vi "Main3.vi"() -> ()   [LabVIEW 2020]
uses:
  <vilib>/userDefined/High Color/IMAQdx.ctl
  <vilib>/vision/Image Controls.llb/IMAQ Image.ctl
  <vilib>/DAQmx/read.llb/DAQmx Read (Analog Wfm 1Chan NSamp).vi
  <vilib>/Utility/error.llb/Error Cluster From Error Code.vi
  <vilib>/DAQmx/miscellaneous.llb/DAQmx Fill In Error Info.vi
  <vilib>/ErrorRing/Error Ring.xnode
  SuportVI2/Message Queue/Message Queue.lvlib
  SuportVI2/User Event - Stop/User Event - Stop.lvlib
  <vilib>/vision/driver/NI_Vision_Acquisition_Software.lvlib
panel:
  out "XY Graph":cluster{dbl[], dbl[]}(graph)
  in  "Data":string="000001"
  in  "Is start":bool
  out "Waveform Graph":waveform(dbl)(graph)
  in  "Aquire Configuration":T1
  in  "Stop Acquire":bool
  in  "Start Acquire":bool
  in  "Stop SinusGen":bool
  in  "Start SinusGen":bool
  in  "Generator Configuration":T1
  out "Image":T2(plugin-control)
  in  "Camera Config":cluster{"Camera Select":T3}={"Camera Select"="cam0"}
  in  "Exit":bool
  in  "Stop Camera":bool
  in  "Start Camera":bool
  out "Status Line":string
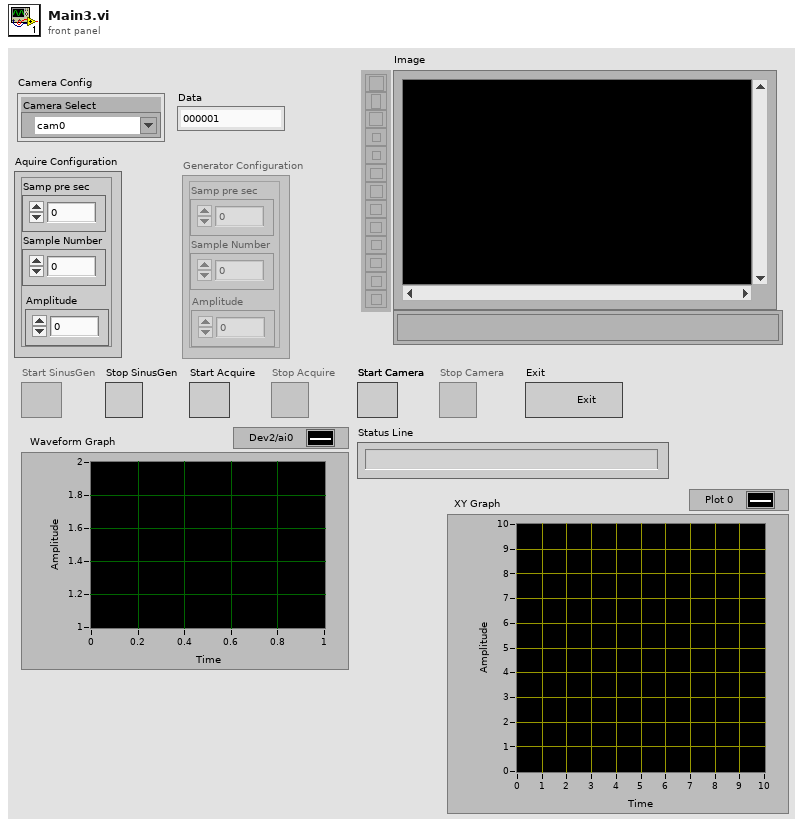
[diagram p1: front panel]
types:
  T1 = cluster{"Sample Number":dbl, "Samp pre sec":i32, "Amplitude":dbl}
  T2 = typedef "IMAQ Image.ctl" = refnum<image>
  T3 = typedef "IMAQdx.ctl" = refnum<k21>
  T4 = cluster{"configuration file path out":path, "DAQmx Task":refnum<k21>, "DAQmx Chanel":cluster{"SampClk.Rate":dbl, "SampQuant.SampPerChan":i32, "Amplitude 2":dbl}}
  T5 = cluster{"DAQmx Task":refnum<k21>, "DAQmx Chanel":cluster{"SampClk.Rate":dbl, "SampQuant.SampPerChan":i32, "Amplitude":dbl}, "DB Data":dbl[][], "DB Cuttoff":dbl[][]}
  T6 = cluster{"Image":cluster{"Image original":T2, "Image copy":T2, "Image Out":T2}, "Session Config":cluster{"Session":T3}, "Data":string}
  T7 = cluster{"Start Camera":refnum<vi>, "Stop Camera":refnum<vi>, "Exit":refnum<vi>, "Camera Conf":refnum<vi>, "Status Line":refnum<vi>, "Status Line Text":string, "Camera Select":refnum<vi>, "Start Acquire":refnum<vi>, "Stop Acquire":refnum<vi>, "Start SinusGen":refnum<vi>, "Stop SinusGen":refnum<vi>, "Generator Configuration":refnum<vi>, "Aquire Configuration":refnum<vi>}
  T8 = cluster{"UI":refnum<queue>, "Camera":refnum<queue>, "Acquire":refnum<queue>, "SinusGen":refnum<queue>}
  T9 = cluster{"SampClk.Rate":dbl, "SampQuant.SampPerChan":i32, dbl}
  T10 = cluster{"SampClk.Rate":dbl, "SampQuant.SampPerChan":i32, "Amplitude":dbl}
  T11 = typedef "Image Type" = u32
  T12 = cluster{"SampClk.Rate":dbl, "SampQuant.SampPerChan":i32, "Amplitude 2":dbl}
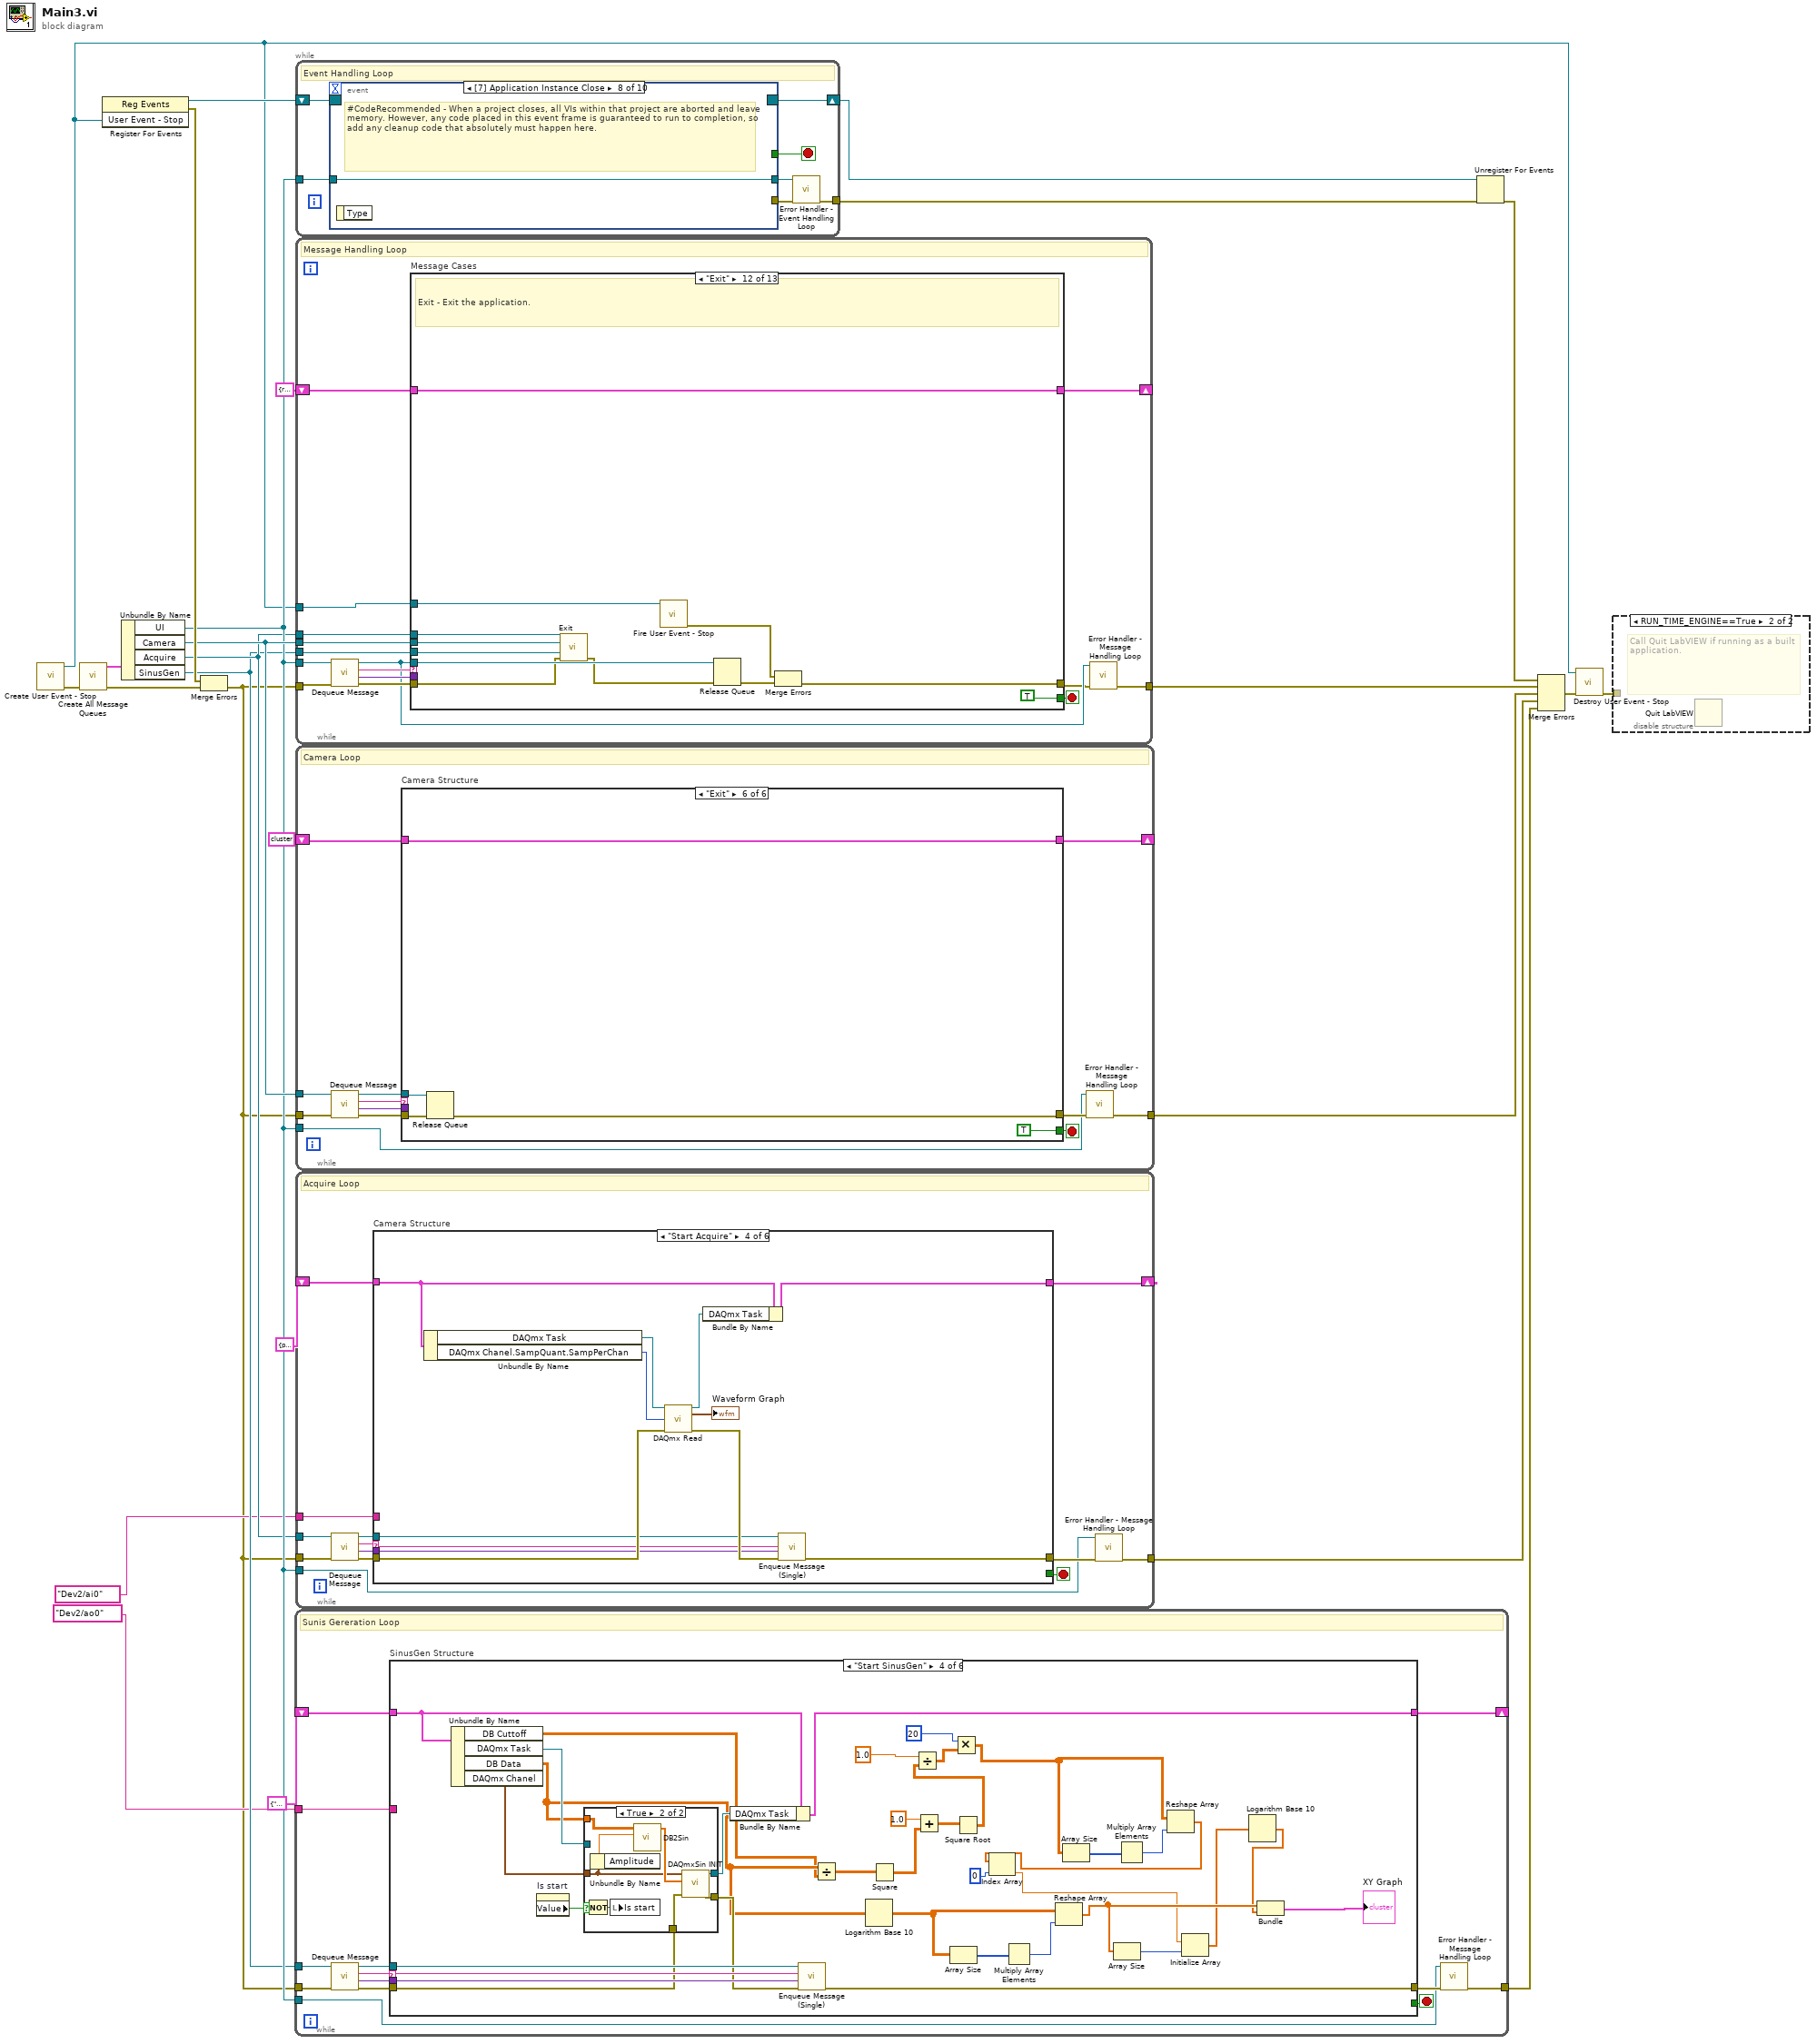
[diagram p0: block diagram]
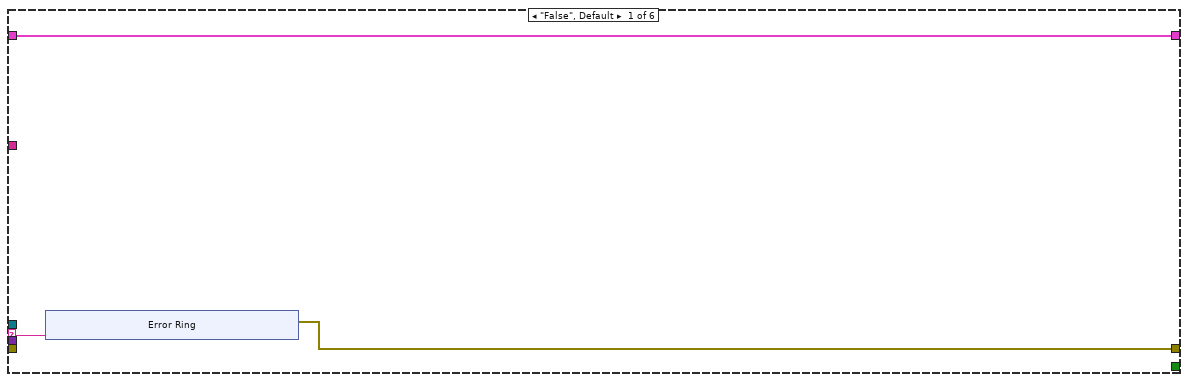
[diagram p2: hidden frame]
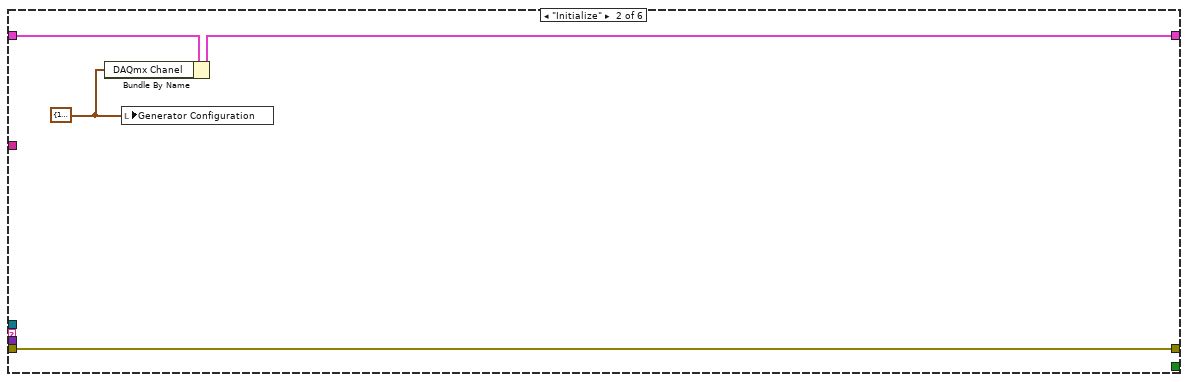
[diagram p3: hidden frame]
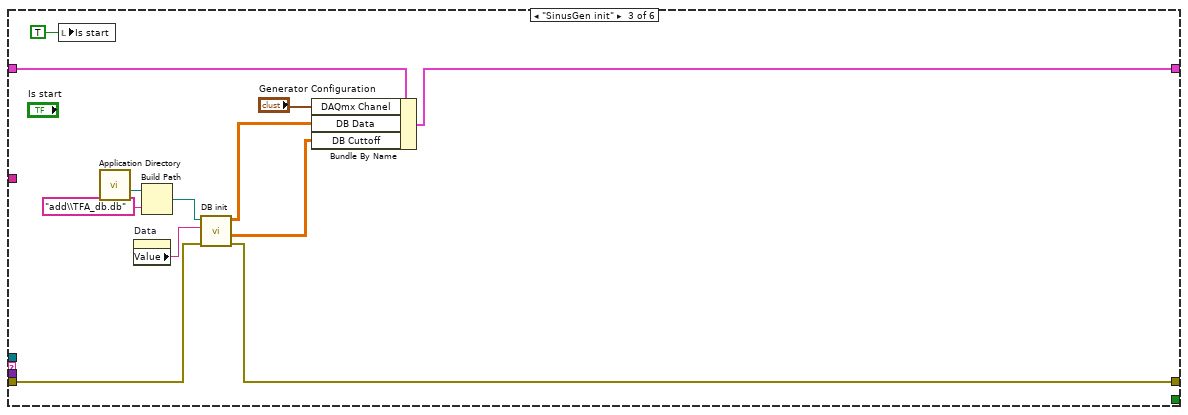
[diagram p4: hidden frame]
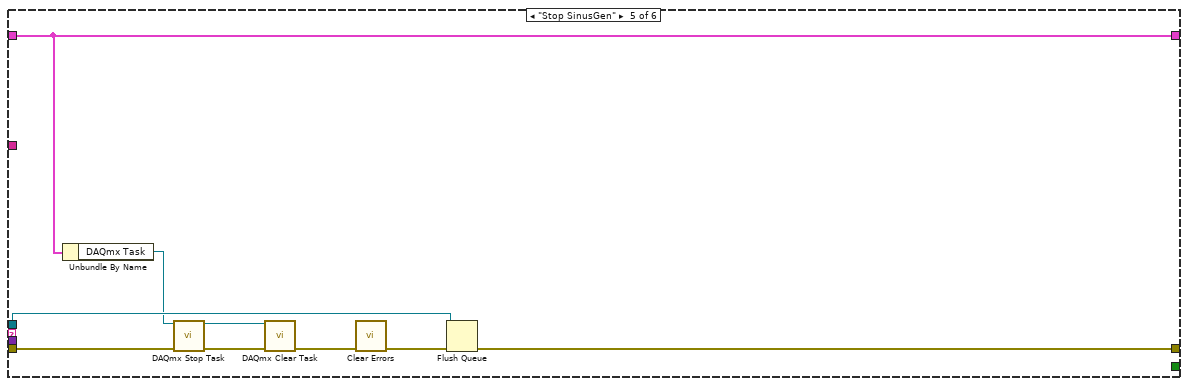
[diagram p6: hidden frame]
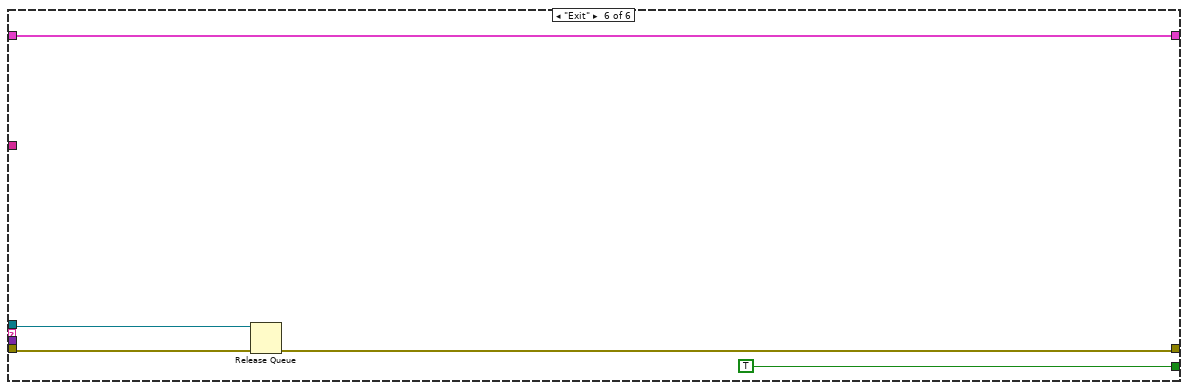
[diagram p7: hidden frame]
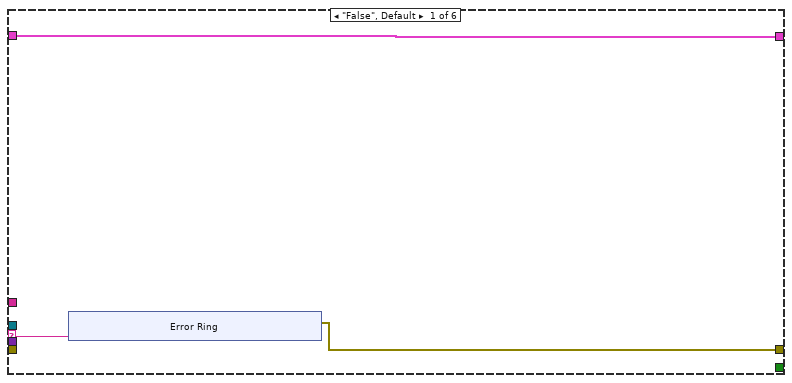
[diagram p8: hidden frame]
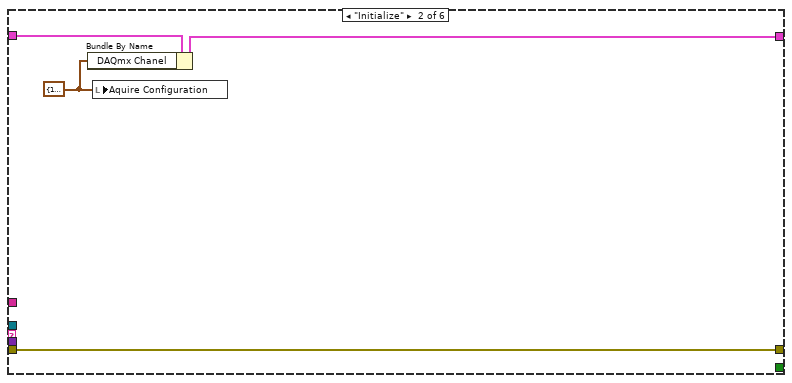
[diagram p9: hidden frame]
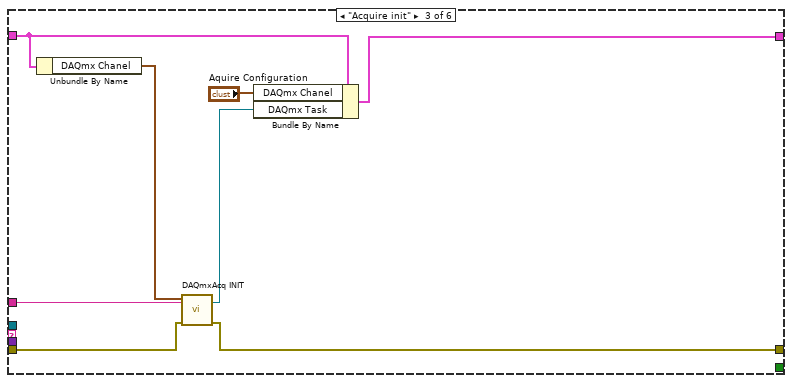
[diagram p10: hidden frame]
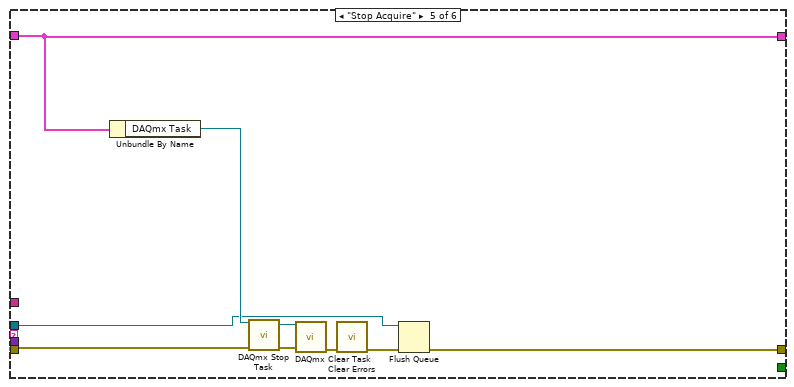
[diagram p11: hidden frame]
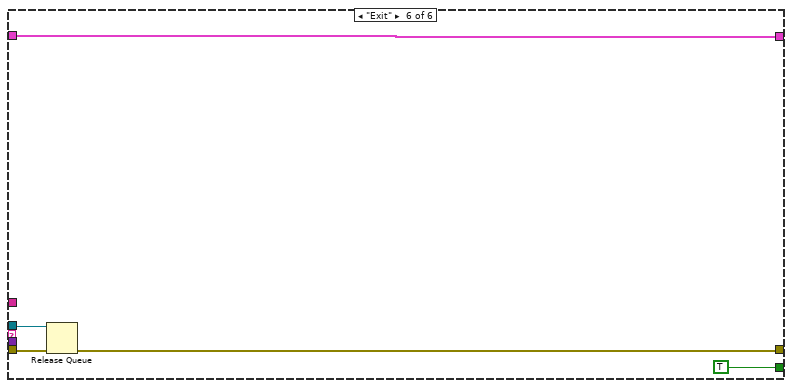
[diagram p12: hidden frame]
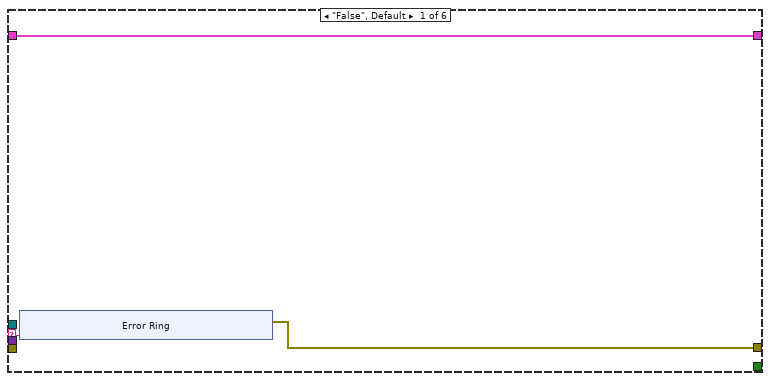
[diagram p13: hidden frame]
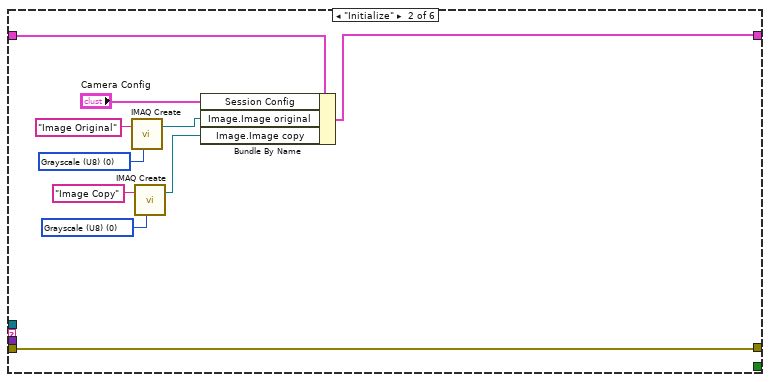
[diagram p14: hidden frame]
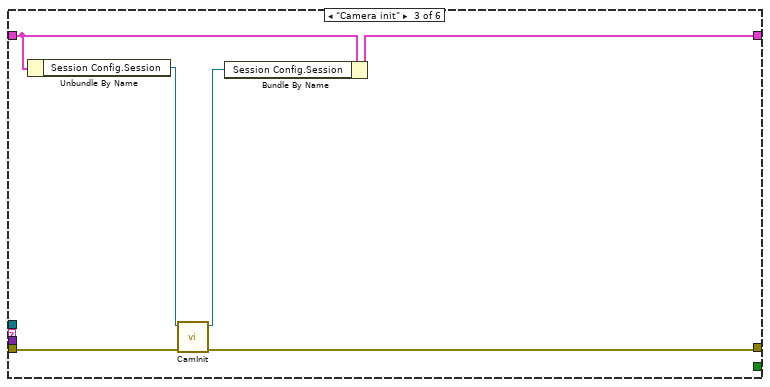
[diagram p15: hidden frame]
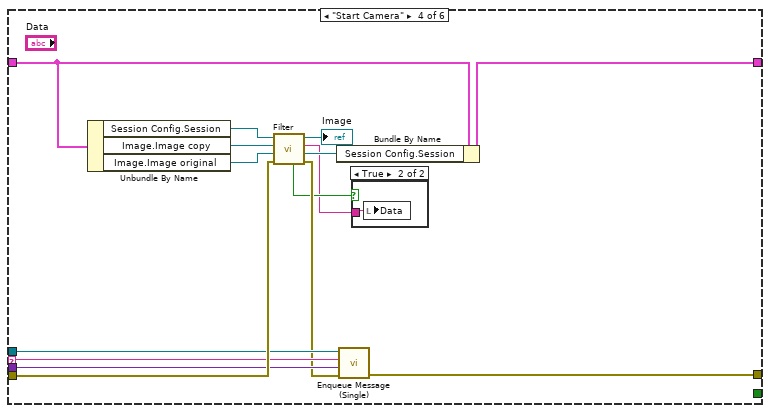
[diagram p16: hidden frame]
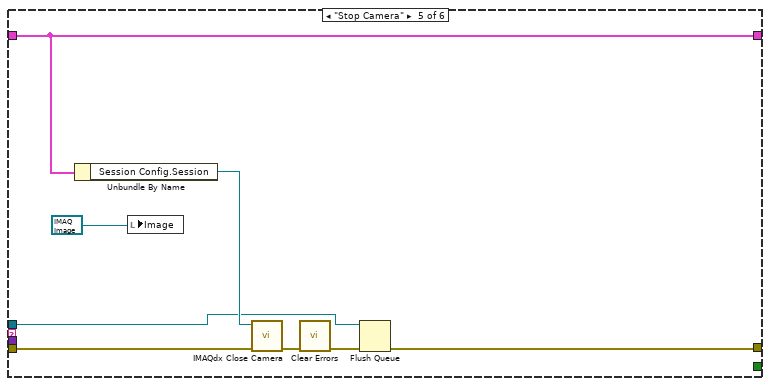
[diagram p18: hidden frame]
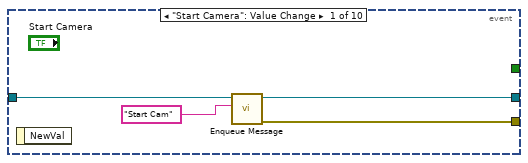
[diagram p20: hidden frame]
diagram:
  n1 = call "Create User Event - Stop.vi"() -> ("error out"=w24:errorcluster, "User Event - Stop"=w10:refnum<user-event>)  [unwired: 10 in]
  n2 = call "Create All Message Queues.vi"("error in (no error)"=w24) -> ("error out"=w26:errorcluster, "Message Queues out"=w14:T8)  [unwired: 9 in]
  n3 = register-events(w10) -> (reference out=w19:refnum<event-registration>, error out=w18:errorcluster)  [unwired: 2 in]
  n4 = Unbundle By Name(w14) -> ("UI"=w12:refnum<queue>, "Camera"=w13:refnum<queue>, "Acquire"=w9:refnum<queue>, "SinusGen"=w8:refnum<queue>)
  n5 = Merge Errors(w18, w26) -> (w4:errorcluster)
  n6 = while {
    tunnel: w12 -> [w27]
    tunnel: w8 -> [w39]
    tunnel: tag "Dev2/ao0" ("physical channels") -> [w38]
    tunnel: w4 -> [w32]
    tunnel: [w28] -> w3
    shift-right: [w31] -> _
    shift-left: T5 {"DAQmx Task"="", "DAQmx Chanel"={"SampClk.Rate"=0.0, "SampQuant.SampPerChan"=0, "Amplitude"=0.0}, "DB Data"=[[5.0]], "DB Cuttoff"=[[50.0]]} -> [w30]
    stop <- w29 stop-if-true
    # "Sunis Gereration Loop"
    n7 = call "Dequeue Message.vi"("error in (no error)"=w32, "Message Queue"=w39) -> ("error out"=w37:errorcluster, "Message Data"=w34:variant, "Message"=w33:string, "dup Message Queue"=w35:refnum<queue>)  [unwired: 6 in]
    n8 = case "SinusGen Structure" shown="\"Start SinusGen\"" w33 {
      selector: w33 -> [w41 _ _ w100 _ _]
      tunnel: [w42 w51 w58 w98 w120 w125] -> w36
      tunnel: w37 -> [_ w51 w63 w93 w114 w124]
      tunnel: w35 -> [_ _ _ w101 w119 w126]
      tunnel: w34 -> [_ _ _ w99 _ _]
      tunnel: [_ _ _ _ _ TRUE] -> w29
      tunnel: [w40 w52 w64 w96 w116 w122] -> w31
      tunnel: w30 -> [w40 w53 w65 w97 w116 w122]
      tunnel: w38 -> [_ _ _ _ _ _]
      frame "False", Default {
        n9 = xnode "Error Ring"("parameter 0"=w41) -> ("error out"=w42:errorcluster)
      }
      frame "Initialize" {
        w50 = T9 {"SampClk.Rate"=1000.0, "SampQuant.SampPerChan"=1000, 5.0} ("DAQmx Chanel")
        n10 = Bundle By Name(cluster=w53, "DAQmx Chanel"=w50) -> (w52:T5)
        n11 = local write "Generator Configuration"(w50) -> ()
      }
      frame "SinusGen init" {
        n12 = local write "Is start"(TRUE ("Boolean")) -> ()
        n13 = call <vilib>:"Application Directory.vi"() -> ("Application Directory"=w62:path)
        n14 = property on="Data" class="Str"() -> ("Value"=w56:string)  [unwired: 2 in, 2 out]
        n15 = Build Path(base path=w62, name or relative path="add\\TFA_db.db") -> (appended path=w60:path)
        n16 = call "DB init.vi"("error in (no error)"=w63, "ID"=w56, "DB path"=w60) -> ("error out"=w58:errorcluster, "DB Cuttoff"=w54:dbl[][], "DB Data"=w55:dbl[][])  [unwired: 6 in]
        n17 = Bundle By Name(cluster=w65, "DAQmx Chanel"="Generator Configuration", "DB Data"=w55, "DB Cuttoff"=w54) -> (w64:T5)
      }
      frame "Start SinusGen" {
        n18 = Unbundle By Name(w97) -> ("DB Cuttoff"=w71:dbl[][], "DAQmx Task"=w91:refnum<k21>, "DB Data"=w76:dbl[][], "DAQmx Chanel"=w95:T10)
        n19 = property on="Is start" class="Bool (strict)"() -> ("Value"=w90:bool)  [unwired: 2 in, 2 out]
        n20 = case shown="True" w90 {
          selector: w90 -> [_ w107]
          tunnel: w76 -> [_ w112]
          tunnel: w95 -> [_ w105]
          tunnel: [w102 w110] -> w94
          tunnel: w93 -> [w103 w109]
          tunnel: [w103 w108] -> w92
          tunnel: w91 -> [w102 _]
          frame False {
          }
          frame True {
            n21 = Not(x=w107) -> (.not. x?=w106:bool)
            n22 = Unbundle By Name(w105) -> ("Amplitude"=w104:dbl)
            n23 = local write "Is start"(w106) -> ()
            n24 = call "DB2Sin.vi"("amplitude"=w104, "DB Data"=w112) -> ("sine wave"=w111:dbl[])  [unwired: 9 in]
            n25 = call "DAQmxSin INIT.vi"("error in"=w109, "sine wave"=w111, "DAQmxChannel"=w105) -> ("error out"=w108:errorcluster, "task out"=w110:refnum<k21>)  [unwired: 7 in]
          }
        }
        n26 = Bundle By Name(cluster=w97, "DAQmx Task"=w94) -> (w96:T5)
        n27 = call "Enqueue Message (Single).vi"("error in (no error)"=w92, "Message Data"=w99, "Message"=w100, "Message Queue"=w101) -> ("error out"=w98:errorcluster)  [unwired: 6 in, 1 out]
        n28 = Divide(x=w76, y=w71) -> (x/y=w87:dbl[][])
        n29 = Logarithm Base 10(1:w76) -> (0:w79:dbl[][])
        n30 = Square(x=w87) -> (x^2=w86:dbl[][])
        n31 = Add(x=1.0, y=w86) -> (x+y=w85:dbl[][])
        n32 = Array Size(array=w79) -> (size(s)=w78:i32[])
        n33 = Square Root(x=w85) -> (sqrt(x)=w84:dbl[][])
        n34 = Divide(x=1.0, y=w84) -> (x/y=w83:dbl[][])
        n35 = Multiply(x=20, y=w83) -> (x*y=w72:dbl[][])
        n36 = Multiply Array Elements(1:w78) -> (0:w77:i32)
        n37 = Reshape Array(w79, w77) -> (w74:dbl[])
        n38 = Array Size(array=w72) -> (size(s)=w81:i32[])
        n39 = Array Size(array=w74) -> (size(s)=w73:i32)
        n40 = Multiply Array Elements(1:w81) -> (0:w80:i32)
        n41 = Reshape Array(w72, w80) -> (w68:dbl[])
        n42 = Index Array(array=w68, index=0 ("index (row)")) -> (element=w70:dbl)
        n43 = Initialize Array(w70, w73) -> (w67:dbl[])
        n44 = Logarithm Base 10(1:w67) -> (0:w69:dbl[])
        n45 = Bundle(w74, w69) -> (→"XY Graph":cluster{dbl[], dbl[]})  [unwired: 1 in]
      }
      frame "Stop SinusGen" {
        n46 = Unbundle By Name(w116) -> ("DAQmx Task"=w115:refnum<k21>)
        n47 = call <vilib>:"DAQmx Stop Task.vi"("task/channels in"=w115, "error in"=w114) -> ("task out"=w118:refnum<k21>, "error out"=w117:errorcluster)  [unwired: 12 in]
        n48 = call <vilib>:"DAQmx Clear Task.vi"("task in"=w118, "error in"=w117) -> ("error out"=w113:errorcluster)  [unwired: 13 in]
        n49 = call <vilib>:"Clear Errors.vi"("error in (no error)"=w113) -> ("error out"=w121:errorcluster)  [unwired: 5 in, 1 out]
        n50 = Flush Queue(queue=w119, error in (no error)=w121) -> (error out=w120:errorcluster)  [unwired: 2 out]
      }
      frame "Exit" {
        n51 = Release Queue(queue=w126, error in (no error)=w124) -> (error out=w125:errorcluster)  [unwired: 1 in, 2 out]
      }
    }
    n52 = call "Error Handler - Message Handling Loop.vi"("error in (no error)"=w36, "Message Queue"=w27) -> ("dup error in"=w28:errorcluster)  [unwired: 8 in, 1 out]
  }
  n53 = while {
    tunnel: w12 -> [w133]
    shift-right: [w131] -> w22
    shift-left: w19 -> [w132]
    tunnel: [w127] -> w20
    stop <- w129 stop-if-true
    # "Event Handling Loop"
    n54 = event shown="[7] Application Instance Close" {
      selector: w132 -> [_ _ _ _ _ _ _ _ _ _]
      dyn-events: [_ _ _ _ _ _ _ _ _ _] -> w131
      timeout: _ -> [_ _ _ _ _ _ _ _ _ _]
      tunnel: [_ _ _ _ _ _ _ _ _ TRUE ("Discard?")] -> w129
      tunnel: w133 -> [w137 w141 w145 w149 w153 w157 w162 w164 w169 w172]
      tunnel: [w134 w138 w142 w146 w150 w154 w161 _ w168 _] -> w130
      tunnel: [w136 w140 w144 w148 w152 w156 w160 w164 w167 w172] -> w128
      event "Start Camera": Value Change {
        n55 = event-data() -> ()  [unwired: 1 in, 1 out]
        n56 = call-poly "Enqueue Message.vi"("Message"="Start Cam", "Message Queue"=w137) -> ("error out"=w134:errorcluster, "dup Message Queue"=w136:refnum<queue>)  [unwired: 8 in]
      }
      event "Start SinusGen": Value Change {
        n57 = event-data() -> ()  [unwired: 1 in, 1 out]
        n58 = call-poly "Enqueue Message.vi"("Message"="Start SinGen", "Message Queue"=w141) -> ("error out"=w138:errorcluster, "dup Message Queue"=w140:refnum<queue>)  [unwired: 8 in]
      }
      event "Start Acquire": Value Change {
        n59 = event-data() -> ()  [unwired: 1 in, 1 out]
        n60 = call-poly "Enqueue Message.vi"("Message"="Start Acq", "Message Queue"=w145) -> ("error out"=w142:errorcluster, "dup Message Queue"=w144:refnum<queue>)  [unwired: 8 in]
      }
      event "Stop Camera": Value Change {
        n61 = event-data() -> ()  [unwired: 1 in, 1 out]
        n62 = call-poly "Enqueue Message.vi"("Message"="Stop Cam", "Message Queue"=w149) -> ("error out"=w146:errorcluster, "dup Message Queue"=w148:refnum<queue>)  [unwired: 8 in]
      }
      event "Stop SinusGen": Value Change {
        n63 = event-data() -> ()  [unwired: 1 in, 1 out]
        n64 = call-poly "Enqueue Message.vi"("Message"="Stop SinGen", "Message Queue"=w153) -> ("error out"=w150:errorcluster, "dup Message Queue"=w152:refnum<queue>)  [unwired: 8 in]
      }
      event "Stop Acquire": Value Change {
        n65 = event-data() -> ()  [unwired: 1 in, 1 out]
        n66 = call-poly "Enqueue Message.vi"("Message"="Stop Acq", "Message Queue"=w157) -> ("error out"=w154:errorcluster, "dup Message Queue"=w156:refnum<queue>)  [unwired: 8 in]
      }
      event Panel Close? {
        # "Send the 'Confirm Quit' message if the user closes the panel of the VI. Discard the event so the 'Confirm Quit' message has a chance to run."
        n67 = event-data() -> ()  [unwired: 1 in, 1 out]
        n68 = call-poly "Enqueue Message.vi"("Priority Message? (F)"=TRUE, "Message"="Confirm Quit", "Message Queue"=w162) -> ("error out"=w161:errorcluster, "dup Message Queue"=w160:refnum<queue>)  [unwired: 7 in]
        n69 = event-data("Discard?"=TRUE) -> ()  [unwired: 1 in, 1 out]
      }
      event Application Instance Close {
        # "#CodeRecommended - When a project closes, all VIs within that project are aborted and leave memory. However, any code placed in this event frame is guaranteed to run to completion, so add any cleanup code that absolutely must happen here."
        n70 = event-data() -> ()  [unwired: 1 in, 1 out]
      }
      event "Exit": Value Change {
        n71 = event-data() -> ()  [unwired: 1 in, 1 out]
        n72 = call-poly "Enqueue Message.vi"("Priority Message? (F)"=TRUE, "Message"="Exit", "Message Queue"=w169) -> ("error out"=w168:errorcluster, "dup Message Queue"=w167:refnum<queue>)  [unwired: 7 in]
      }
      event User Event {
        # "The Message Handling Loop processed an \"Exit\" message, which fired this event to stop the Event Handling Loop."
        n73 = event-data() -> ()  [unwired: 1 in, 1 out]
        n74 = local write "Status Line"("Exiting application" ("VI Stopped")) -> ()
      }
    }
    n75 = call "Error Handler - Event Handling Loop.vi"("error in (no error)"=w130, "Message Queue"=w128) -> ("dup error in"=w127:errorcluster)  [unwired: 8 in, 1 out]
  }
  n76 = while {
    tunnel: w12 -> [w180]
    shift-right: [w186] -> _
    shift-left: T7 {"Start Camera"=refnum, "Stop Camera"=refnum, "Exit"=refnum, "Camera Conf"=refnum, "Status Line"=refnum, "Status Line Text"="", "Camera Select"=refnum, "Start Acquire"=refnum, "Stop Acquire"=refnum, "Start SinusGen"=refnum, "Stop SinusGen"=refnum, "Generator Configuration"=refnum, "Aquire Configuration"=refnum} -> [w187]
    tunnel: w10 -> [w184]
    tunnel: w4 -> [w173]
    tunnel: [w178] -> w25
    tunnel: w13 -> [w176]
    tunnel: w9 -> [w175]
    tunnel: w8 -> [w174]
    stop <- w185 stop-if-true
    # "Message Handling Loop"
    n77 = call "Dequeue Message.vi"("error in (no error)"=w173, "Message Queue"=w180) -> ("error out"=w183:errorcluster, "Message Data"=w181:variant, "Message"=w182:string, "dup Message Queue"=w179:refnum<queue>)  [unwired: 6 in]
    n78 = case "Message Cases" shown="\"Exit\"" w182 {
      selector: w182 -> [_ _ _ _ _ _ _ _ _ _ _ _ w355]
      tunnel: w179 -> [w207 w226 w243 w260 w280 w298 w316 _ _ w335 _ w354 _]
      tunnel: w183 -> [w212 w223 w241 w258 w277 w295 w313 w323 w332 w339 w342 w344 _]
      tunnel: [w213 w230 w247 w264 w282 w300 w318 w324 w326 w337 w340 w351 w356] -> w177
      tunnel: w187 -> [w211 w221 w239 w256 w265 w284 w302 w325 w331 w338 w341 w348 w357]
      tunnel: [w210 w221 w239 w256 w265 w284 w302 w325 w331 w338 w341 w348 w357] -> w186
      tunnel: [_ _ _ _ _ _ _ _ _ _ _ TRUE _] -> w185
      tunnel: w181 -> [_ _ _ _ _ _ _ w322 w330 _ _ _ _]
      tunnel: w184 -> [_ _ _ _ _ _ _ _ _ _ _ w350 _]
      tunnel: w176 -> [_ w225 _ _ w275 _ _ _ _ _ _ w346 _]
      tunnel: w175 -> [_ _ _ w248 _ _ w301 _ _ _ _ w347 _]
      tunnel: w174 -> [_ _ w231 _ _ w283 _ _ _ _ _ w345 _]
      frame "Initialize" {
        w206 = "Initialization Completed" ("Initial Message")
        # "Initialize - All initialization work should take place in this message, since other loops can potentially enqueue messages that execute immediately after this one."
        n79 = control-ref of="Start Camera"() -> (w188:refnum<vi>)
        n80 = control-ref of="Stop Camera"() -> (w203:refnum<vi>)
        n81 = control-ref of="Exit"() -> (w194:refnum<vi>)
        n82 = control-ref of="Start Acquire"() -> (w192:refnum<vi>)
        n83 = control-ref of="Stop Acquire"() -> (w198:refnum<vi>)
        n84 = control-ref of="Start SinusGen"() -> (w191:refnum<vi>)
        n85 = control-ref of="Stop SinusGen"() -> (w197:refnum<vi>)
        n86 = control-ref of="Camera Config"() -> (w193:refnum<vi>)
        n87 = control-ref of="Generator Configuration"() -> (w190:refnum<vi>)
        n88 = control-ref of="Aquire Configuration"() -> (w189:refnum<vi>)
        n89 = control-ref of="Status Line"() -> (w209:refnum<vi>)
        n90 = Bundle By Name(cluster=w211, "Start Camera"=w188, "Stop Camera"=w203, "Status Line"=w209, "Exit"=w194, "Status Line Text"=w206, "Camera Select"=w193, "Start Acquire"=w192, "Stop Acquire"=w198, "Start SinusGen"=w191, "Stop SinusGen"=w197, "Generator Configuration"=w190, "Aquire Configuration"=w189) -> (w210:T7)
        n91 = call-poly "Enqueue Message.vi"("error in (no error)"=w212, "Message Data"=w206, "Message"="Update Display", "Message Queue"=w207) -> ("error out"=w213:errorcluster)  [unwired: 6 in, 1 out]
        n92 = Build Array(w203) -> (w204:refnum<vi>[])
        n93 = Build Array(w198) -> (w201:refnum<vi>[])
        n94 = Build Array(w197) -> (w199:refnum<vi>[])
        n95 = call "Set Enable State on Multiple Controls.vi"("Enable?"=FALSE, "Controls"=w204) -> ()  [unwired: 10 in]
        n96 = call "Set Enable State on Multiple Controls.vi"("Enable?"=FALSE, "Controls"=w201) -> ()  [unwired: 10 in]
        n97 = call "Set Enable State on Multiple Controls.vi"("Enable?"=FALSE, "Controls"=w199) -> ()  [unwired: 10 in]
        n98 = Build Array(w188, w194, w193, w192, w191, w190, w189) -> (w196:refnum<vi>[])
        n99 = call "Set Enable State on Multiple Controls.vi"("Enable?"=TRUE, "Controls"=w196) -> ()  [unwired: 10 in]
      }
      frame "Start Cam" {
        w224 = string[] ["Camera init", "Start Camera"]  # Elementy kolejki
        # "Something - Replace this message with functionality for your own application."
        n100 = Unbundle By Name(w221) -> ("Start Camera"=w215:refnum<vi>, "Camera Conf"=w216:refnum<vi>, "Stop Camera"=w217:refnum<vi>)
        n101 = call "Message Queue (Array).vi"("error in (no error)"=w223, "Message Array"=w224, "Message Queue"=w225) -> ("error out"=w222:errorcluster)  [unwired: 7 in, 1 out]
        n102 = Build Array(w215, w216) -> (w220:refnum<vi>[])
        n103 = Build Array(w217) -> (w219:refnum<vi>[])
        n104 = call "Set Enable State on Multiple Controls.vi"("Enable?"=FALSE, "Controls"=w220) -> ()  [unwired: 10 in]
        n105 = call "Set Enable State on Multiple Controls.vi"("Enable?"=TRUE, "Controls"=w219) -> ()  [unwired: 10 in]
        n106 = call-poly "Enqueue Message.vi"("error in (no error)"=w222, "Message Data"="Starting Camera..." ("\"Do Something\" button pressed"), "Message"="Update Display", "Message Queue"=w226) -> ("error out"=w229:errorcluster)  [unwired: 6 in, 1 out]
        n107 = Merge Errors(w229) -> (w230:errorcluster)
      }
      frame "Start SinGen" {
        w242 = string[] ["SinusGen init", "Start SinusGen"]  # Elementy kolejki
        # "Something - Replace this message with functionality for your own application."
        n108 = Unbundle By Name(w239) -> ("Start SinusGen"=w233:refnum<vi>, "Generator Configuration"=w234:refnum<vi>, "Stop SinusGen"=w235:refnum<vi>)
        n109 = call "Message Queue (Array).vi"("error in (no error)"=w241, "Message Array"=w242, "Message Queue"=w231) -> ("error out"=w240:errorcluster)  [unwired: 7 in, 1 out]
        n110 = Build Array(w233, w234) -> (w238:refnum<vi>[])
        n111 = Build Array(w235) -> (w237:refnum<vi>[])
        n112 = call "Set Enable State on Multiple Controls.vi"("Enable?"=FALSE, "Controls"=w238) -> ()  [unwired: 10 in]
        n113 = call "Set Enable State on Multiple Controls.vi"("Enable?"=TRUE, "Controls"=w237) -> ()  [unwired: 10 in]
        n114 = call-poly "Enqueue Message.vi"("error in (no error)"=w240, "Message Data"="Starting SinusGen..." ("\"Do Something\" button pressed"), "Message"="Update Display", "Message Queue"=w243) -> ("error out"=w246:errorcluster)  [unwired: 6 in, 1 out]
        n115 = Merge Errors(w246) -> (w247:errorcluster)
      }
      frame "Start Acq" {
        w259 = string[] ["Acquire init", "Start Acquire"]  # Elementy kolejki
        # "Something - Replace this message with functionality for your own application."
        n116 = Unbundle By Name(w256) -> ("Start Acquire"=w250:refnum<vi>, "Aquire Configuration"=w251:refnum<vi>, "Stop Acquire"=w252:refnum<vi>)
        n117 = call "Message Queue (Array).vi"("error in (no error)"=w258, "Message Array"=w259, "Message Queue"=w248) -> ("error out"=w257:errorcluster)  [unwired: 7 in, 1 out]
        n118 = Build Array(w250, w251) -> (w255:refnum<vi>[])
        n119 = Build Array(w252) -> (w254:refnum<vi>[])
        n120 = call "Set Enable State on Multiple Controls.vi"("Enable?"=FALSE, "Controls"=w255) -> ()  [unwired: 10 in]
        n121 = call "Set Enable State on Multiple Controls.vi"("Enable?"=TRUE, "Controls"=w254) -> ()  [unwired: 10 in]
        n122 = call-poly "Enqueue Message.vi"("error in (no error)"=w257, "Message Data"="Starting Acquire..." ("\"Do Something\" button pressed"), "Message"="Update Display", "Message Queue"=w260) -> ("error out"=w263:errorcluster)  [unwired: 6 in, 1 out]
        n123 = Merge Errors(w263) -> (w264:errorcluster)
      }
      frame "Stop Cam" {
        # "Something Else - Replace this message with functionality for your own application."
        n124 = Unbundle By Name(w265) -> ("Start Camera"=w267:refnum<vi>, "Camera Conf"=w268:refnum<vi>, "Stop Camera"=w269:refnum<vi>)
        n125 = call-poly "Enqueue Message.vi"("Priority Message? (F)"=TRUE, "error in (no error)"=w277, "Message"="Stop Camera", "Message Queue"=w275) -> ("error out"=w276:errorcluster)  [unwired: 6 in, 1 out]
        n126 = Build Array(w267, w268) -> (w272:refnum<vi>[])
        n127 = Build Array(w269) -> (w271:refnum<vi>[])
        n128 = call-poly "Enqueue Message.vi"("error in (no error)"=w276, "Message Data"="Camera Stopped" ("\"Do Something Else\" button pressed"), "Message"="Update Display", "Message Queue"=w280) -> ("error out"=w281:errorcluster)  [unwired: 6 in, 1 out]
        n129 = call "Set Enable State on Multiple Controls.vi"("Enable?"=TRUE, "Controls"=w272) -> ()  [unwired: 10 in]
        n130 = call "Set Enable State on Multiple Controls.vi"("Enable?"=FALSE, "Controls"=w271) -> ()  [unwired: 10 in]
        n131 = Merge Errors(w281) -> (w282:errorcluster)
      }
      frame "Stop SinGen" {
        # "Something Else - Replace this message with functionality for your own application."
        n132 = Unbundle By Name(w284) -> ("Start SinusGen"=w286:refnum<vi>, "Generator Configuration"=w287:refnum<vi>, "Stop SinusGen"=w288:refnum<vi>)
        n133 = call-poly "Enqueue Message.vi"("Priority Message? (F)"=TRUE, "error in (no error)"=w295, "Message"="Stop SinusGen", "Message Queue"=w283) -> ("error out"=w294:errorcluster)  [unwired: 6 in, 1 out]
        n134 = Build Array(w286, w287) -> (w291:refnum<vi>[])
        n135 = Build Array(w288) -> (w290:refnum<vi>[])
        n136 = call "Set Enable State on Multiple Controls.vi"("Enable?"=TRUE, "Controls"=w291) -> ()  [unwired: 10 in]
        n137 = call "Set Enable State on Multiple Controls.vi"("Enable?"=FALSE, "Controls"=w290) -> ()  [unwired: 10 in]
        n138 = call-poly "Enqueue Message.vi"("error in (no error)"=w294, "Message Data"="SinusGen Stopped" ("\"Do Something Else\" button pressed"), "Message"="Update Display", "Message Queue"=w298) -> ("error out"=w299:errorcluster)  [unwired: 6 in, 1 out]
        n139 = Merge Errors(w299) -> (w300:errorcluster)
      }
      frame "Stop Acq" {
        # "Something Else - Replace this message with functionality for your own application."
        n140 = Unbundle By Name(w302) -> ("Start Acquire"=w304:refnum<vi>, "Aquire Configuration"=w305:refnum<vi>, "Stop Acquire"=w306:refnum<vi>)
        n141 = call-poly "Enqueue Message.vi"("Priority Message? (F)"=TRUE, "error in (no error)"=w313, "Message"="Stop Acquire", "Message Queue"=w301) -> ("error out"=w312:errorcluster)  [unwired: 6 in, 1 out]
        n142 = Build Array(w304, w305) -> (w309:refnum<vi>[])
        n143 = Build Array(w306) -> (w308:refnum<vi>[])
        n144 = call "Set Enable State on Multiple Controls.vi"("Enable?"=TRUE, "Controls"=w309) -> ()  [unwired: 10 in]
        n145 = call "Set Enable State on Multiple Controls.vi"("Enable?"=FALSE, "Controls"=w308) -> ()  [unwired: 10 in]
        n146 = call-poly "Enqueue Message.vi"("error in (no error)"=w312, "Message Data"="Acquire Stopped" ("\"Do Something Else\" button pressed"), "Message"="Update Display", "Message Queue"=w316) -> ("error out"=w317:errorcluster)  [unwired: 6 in, 1 out]
        n147 = Merge Errors(w317) -> (w318:errorcluster)
      }
      frame "Update Display" {
        # "Update Display - Convert the message data to a string to display in the Data Display indicator."
        n148 = Variant To Data(error in=w323, type="", Variant=w322) -> (data=→"Status Line":string, error out=w320:errorcluster)
        n149 = Merge Errors(w320) -> (w324:errorcluster)
      }
      frame "Error" {
        # "Error - Display an error dialog. This message is sent by the \"Error Handler\" VIs at the end of other loops in this application."
        n150 = Variant To Data(error in=w332, type=errorcluster {"status"=FALSE, "code"=0, "source"=""} ("error constant"), Variant=w330) -> (data=w328:errorcluster, error out=w327:errorcluster)
        n151 = call <vilib>:"Simple Error Handler.vi"("error in (no error)"=w328) -> ()  [unwired: 4 in, 5 out]
        n152 = Merge Errors(w327) -> (w326:errorcluster)
      }
      frame "Confirm Quit" {
        # "Confirm Quit - Message that can confirm whether or not the user wants to exit the application."
        n153 = call-poly "Enqueue Message.vi"("Priority Message? (F)"=TRUE, "error in (no error)"=w339, "Message"="Exit", "Message Queue"=w335) -> ("error out"=w336:errorcluster)  [unwired: 6 in, 1 out]
        n154 = Merge Errors(w336) -> (w337:errorcluster)
      }
      frame "---Copy This Frame---" {
        # "Duplicate this frame when creating new messages.  Change this comment in the duplicated frame to describe this message."
        n155 = Merge Errors(w342) -> (w340:errorcluster)
      }
      frame "Exit" {
        # "Exit - Exit the application."
        n156 = call "Exit.vi"("error in"=w344, "Message Sin"=w345, "Message Acq"=w347, "Message Cam"=w346) -> ("error out"=w343:errorcluster)  [unwired: 7 in]
        n157 = call "Fire User Event - Stop.vi"("User Event - Stop"=w350) -> ("error out"=w349:errorcluster)  [unwired: 10 in]
        n158 = Release Queue(queue=w354, error in (no error)=w343) -> (error out=w352:errorcluster)  [unwired: 1 in, 2 out]
        n159 = Merge Errors(w349, w352) -> (w351:errorcluster)
      }
      frame Default {
        # "'Default' case only runs if there is a message that isn't defined in any of the other cases.  Output a programming error."
        n160 = xnode "Error Ring"("parameter 0"=w355) -> ("error out"=w356:errorcluster)
      }
    }
    n161 = call "Error Handler - Message Handling Loop.vi"("error in (no error)"=w177, "Message Queue"=w179) -> ("dup error in"=w178:errorcluster)  [unwired: 8 in, 1 out]
  }
  n162 = while {
    shift-right: [w368] -> _
    shift-left: T6 {"Image"={"Image original"=refnum, "Image copy"=refnum, "Image Out"=refnum}, "Session Config"={"Session"=""}, "Data"=""} ("Camera conf Cluster") -> [w371]
    tunnel: [w376] -> w16
    tunnel: w4 -> [w375]
    tunnel: w12 -> [w372]
    tunnel: w13 -> [w370]
    stop <- w366 stop-if-true
    # "Camera Loop"
    n163 = call "Dequeue Message.vi"("error in (no error)"=w375, "Message Queue"=w370) -> ("error out"=w374:errorcluster, "Message Data"=w367:variant, "Message"=w365:string, "dup Message Queue"=w369:refnum<queue>)  [unwired: 6 in]
    n164 = case "Camera Structure" shown="\"Exit\"" w365 {
      selector: w365 -> [w377 _ _ w409 _ _]
      tunnel: [w379 w396 w399 w406 w421 w429] -> w373
      tunnel: w374 -> [_ w396 w400 w417 w426 w428]
      tunnel: w371 -> [w378 w394 w398 w413 w425 w431]
      tunnel: w369 -> [_ _ _ w410 w420 w430]
      tunnel: [w378 w393 w397 w411 w425 w431] -> w368
      tunnel: w367 -> [_ _ _ w408 _ _]
      tunnel: [_ _ _ _ _ TRUE] -> w366
      frame "False", Default {
        n165 = xnode "Error Ring"("parameter 0"=w377) -> ("error out"=w379:errorcluster)
      }
      frame "Initialize" {
        w388 = T11 0 items=["Grayscale (U8)", "Grayscale (I16)", "Grayscale (SGL)", "Complex (CSG)", "RGB (U32)", "HSL (U32)", "RGB (U64)", "Grayscale (U16)"] ("Image Type")
        w391 = T11 0 items=["Grayscale (U8)", "Grayscale (I16)", "Grayscale (SGL)", "Complex (CSG)", "RGB (U32)", "HSL (U32)", "RGB (U64)", "Grayscale (U16)"] ("Image Type")
        n166 = call "IMAQ Create"("Image Name"="Image Original", "Image Type"=w388) -> ("New Image"=w387:T2)  [unwired: 3 in, 1 out]
        n167 = call "IMAQ Create"("Image Name"="Image Copy", "Image Type"=w391) -> ("New Image"=w390:T2)  [unwired: 3 in, 1 out]
        n168 = Bundle By Name(cluster=w394, "Session Config"="Camera Config", "Image.Image original"=w387, "Image.Image copy"=w390) -> (w393:T6)
      }
      frame "Camera init" {
        n169 = Unbundle By Name(w398) -> ("Session Config.Session"=w402:T3)
        n170 = call "CamInit.vi"("error in (no error)"=w400, "Refnum in"=w402) -> ("error out"=w399:errorcluster, "Refnum out"=w401:T3)  [unwired: 8 in]
        n171 = Bundle By Name(cluster=w398, "Session Config.Session"=w401) -> (w397:T6)
      }
      frame "Start Camera" {
        n172 = Unbundle By Name(w413) -> ("Session Config.Session"=w416:T3, "Image.Image copy"=w415:T2, "Image.Image original"=w414:T2)
        n173 = call "Filter.vi"("error in"=w417, "Image original"=w414, "Image copy"=w415, "Session Config"=w416) -> ("error out"=w407:errorcluster, "Session Out"=w412:T3, "Data"=w403:string, "Image Out"=→"Image":T2, "Found?"=w404:bool)  [unwired: 3 in]
        n174 = Bundle By Name(cluster=w413, "Session Config.Session"=w412) -> (w411:T6)
        n175 = call "Enqueue Message (Single).vi"("error in (no error)"=w407, "Message Data"=w408, "Message"=w409, "Message Queue"=w410) -> ("error out"=w406:errorcluster)  [unwired: 6 in, 1 out]
        n176 = case shown="True" w404 {
          tunnel: w403 -> [_ w418]
          frame False {
          }
          frame True {
            n177 = local write "Data"(w418) -> ()
          }
        }
      }
      frame "Stop Camera" {
        n178 = Unbundle By Name(w425) -> ("Session Config.Session"=w424:T3)
        n179 = local write "Image"(T2 refnum ("Image")) -> ()
        n180 = call <vilib>:"IMAQdx Close Camera.vi"("error in"=w426, "Session In"=w424) -> ("error out"=w422:errorcluster)  [unwired: 9 in]
        n181 = call <vilib>:"Clear Errors.vi"("error in (no error)"=w422) -> ("error out"=w423:errorcluster)  [unwired: 5 in, 1 out]
        n182 = Flush Queue(queue=w420, error in (no error)=w423) -> (error out=w421:errorcluster)  [unwired: 2 out]
      }
      frame "Exit" {
        n183 = Release Queue(queue=w430, error in (no error)=w428) -> (error out=w429:errorcluster)  [unwired: 1 in, 2 out]
      }
    }
    n184 = call "Error Handler - Message Handling Loop.vi"("error in (no error)"=w373, "Message Queue"=w372) -> ("dup error in"=w376:errorcluster)  [unwired: 8 in, 1 out]
  }
  n185 = while {
    shift-right: [w436] -> _
    shift-left: T4 {"configuration file path out"=path "", "DAQmx Task"="", "DAQmx Chanel"={"SampClk.Rate"=0.0, "SampQuant.SampPerChan"=0, "Amplitude 2"=0.0}} -> [w435]
    tunnel: [w433] -> w7
    tunnel: w9 -> [w442]
    tunnel: w4 -> [w437]
    tunnel: w12 -> [w432]
    tunnel: tag "Dev2/ai0" ("physical channels") -> [w434]
    stop <- w439 stop-if-true
    # "Acquire Loop"
    n186 = call "Dequeue Message.vi"("error in (no error)"=w437, "Message Queue"=w442) -> ("error out"=w444:errorcluster, "Message Data"=w440:variant, "Message"=w438:string, "dup Message Queue"=w441:refnum<queue>)  [unwired: 6 in]
    n187 = case "Camera Structure" shown="\"Start Acquire\"" w438 {
      selector: w438 -> [w446 _ _ w471 _ _]
      tunnel: [w447 w456 w459 w473 w482 w491] -> w443
      tunnel: w444 -> [_ w456 w462 w474 w481 w490]
      tunnel: w441 -> [_ _ _ w470 w479 w492]
      tunnel: w440 -> [_ _ _ w472 _ _]
      tunnel: [_ _ _ _ _ TRUE] -> w439
      tunnel: [w445 w457 w465 w476 w483 w488] -> w436
      tunnel: w435 -> [w445 w458 w466 w477 w483 w488]
      tunnel: w434 -> [_ _ w460 _ _ _]
      frame "False", Default {
        n188 = xnode "Error Ring"("parameter 0"=w446) -> ("error out"=w447:errorcluster)
      }
      frame "Initialize" {
        w455 = T10 {"SampClk.Rate"=1000.0, "SampQuant.SampPerChan"=1000, "Amplitude"=5.0} ("DAQmx Chanel")
        n189 = Bundle By Name(cluster=w458, "DAQmx Chanel"=w455) -> (w457:T4)
        n190 = local write "Aquire Configuration"(w455) -> ()
      }
      frame "Acquire init" {
        n191 = Unbundle By Name(w466) -> ("DAQmx Chanel"=w463:T12)
        n192 = call "DAQmxAcq INIT.vi"("physical channels"=w460, "error in"=w462, "DAQmxChannel"=w463) -> ("error out"=w459:errorcluster, "task out"=w461:refnum<k21>)  [unwired: 7 in]
        n193 = Bundle By Name(cluster=w466, "DAQmx Chanel"="Aquire Configuration", "DAQmx Task"=w461) -> (w465:T4)
      }
      frame "Start Acquire" {
        n194 = Unbundle By Name(w477) -> ("DAQmx Task"=w469:refnum<k21>, "DAQmx Chanel.SampQuant.SampPerChan"=w475:i32)
        n195 = call-poly <vilib>:"DAQmx Read.vi"("task/channels in"=w469, "number of samples per channel"=w475, "error in"=w474) -> ("task out"=w468:refnum<k21>, "data"=→"Waveform Graph":waveform(dbl), "error out"=w478:errorcluster)  [unwired: 10 in]
        n196 = Bundle By Name(cluster=w477, "DAQmx Task"=w468) -> (w476:T4)
        n197 = call "Enqueue Message (Single).vi"("error in (no error)"=w478, "Message Data"=w472, "Message"=w471, "Message Queue"=w470) -> ("error out"=w473:errorcluster)  [unwired: 6 in, 1 out]
      }
      frame "Stop Acquire" {
        n198 = Unbundle By Name(w483) -> ("DAQmx Task"=w480:refnum<k21>)
        n199 = call <vilib>:"DAQmx Stop Task.vi"("task/channels in"=w480, "error in"=w481) -> ("task out"=w485:refnum<k21>, "error out"=w484:errorcluster)  [unwired: 12 in]
        n200 = call <vilib>:"DAQmx Clear Task.vi"("task in"=w485, "error in"=w484) -> ("error out"=w486:errorcluster)  [unwired: 13 in]
        n201 = call <vilib>:"Clear Errors.vi"("error in (no error)"=w486) -> ("error out"=w487:errorcluster)  [unwired: 5 in, 1 out]
        n202 = Flush Queue(queue=w479, error in (no error)=w487) -> (error out=w482:errorcluster)  [unwired: 2 out]
      }
      frame "Exit" {
        n203 = Release Queue(queue=w492, error in (no error)=w490) -> (error out=w491:errorcluster)  [unwired: 1 in, 2 out]
      }
    }
    n204 = call "Error Handler - Message Handling Loop.vi"("error in (no error)"=w443, "Message Queue"=w432) -> ("dup error in"=w433:errorcluster)  [unwired: 8 in, 1 out]
  }
  n205 = Unregister For Events(event registration refnum=w22, error in=w20) -> (error out=w23:errorcluster)
  n206 = Merge Errors(w23, w25, w16, w7, w3) -> (w1:errorcluster)
  n207 = call "Destroy User Event - Stop.vi"("error in (no error)"=w1, "User Event - Stop"=w10) -> ("error out"=w21:errorcluster)  [unwired: 9 in]
  n208 = disable-structure shown="RUN_TIME_ENGINE==True" {
    disable-tunnel: w21 -> [_ _]
    frame condition #0 (active) {
    }
    frame condition #1 {
      # "Call Quit LabVIEW if running as a built application."
      n209 = Quit LabVIEW() -> ()  [unwired: 1 in]
    }
  }
